vi "Do.vi"(8 "error in":errorcluster, 10 "Actor in":refnum<class "Actor.lvclass">, 11 "Send Shutdown MSG":refnum<class "Send Shutdown MSG.lvclass">) -> (0 "error out":errorcluster, 2 "Actor out":refnum<class "Actor.lvclass">)   [LabVIEW 2016, in "SuperActor.lvlib" / "Send Shutdown MSG.lvclass"]
doc: "(<B>Filename</B>: Actor Framework.lvlib:Message.lvclass:Do.vi)\n\nDefines what a message does when it is received by an actor. Generally, a message instructs an actor to invoke one of its methods. By default, this method does nothing. A child class must override it to define behavior. Create a child class by using the Actor Framework Message Maker dialog box."
uses:
  Send Shutdown MSG.lvclass
  <vilib>/ActorFramework/Actor/Actor.lvclass
  SuperActor.lvclass
  C:/Program Files (x86)/National Instruments/LabVIEW 2016/vi.lib/ActorFramework/Actor/Actor.lvclass
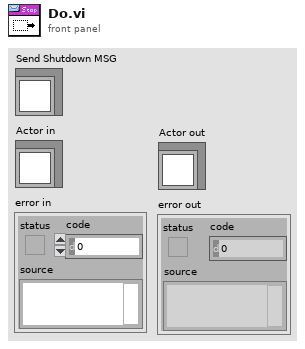
[diagram p1: front panel]
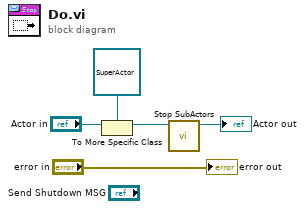
[diagram p0: block diagram]
diagram:
  n1 = To More Specific Class(target class=refnum<class "SuperActor.lvclass"> refnum ("Untitled Library 2:SuperActor"), reference="Actor in") -> (specific class reference=w2:refnum<class "SuperActor.lvclass">)  [unwired: 1 in, 1 out]
  n2 = call "Stop SubActors.vi"("SuperActor in"=w2) -> ("SuperActor out"=→"Actor out":refnum<class "SuperActor.lvclass">)  [unwired: 10 in]
  "error out" <- "error in"
